vi "SPARK Set Sensor Position.vi"(7 "Sensor (Primary Encoder)":enum16{"Primary Encoder", "Alt/Ext Encoder"}(ring), 8 "error in":errorcluster, 10 "Position":dbl, 11 "MotorControlDeviceRef":T1={"DeviceStatus"={"status"=FALSE, "code"=0, "source"=""}, "Type"=enum."PWM", "PWM"={"PWM Channel"=enum."Invalid", "DeadBand"={"Name"="", "maxPositivePwm"=0, "minPositivePwm"=0, "centerPwm"=0, "maxNegativePwm"=0, "minNegativePwm"=0, "angularRange"=0}}, "CAN"={"Device Number"=0, "SetOutput VI Ref"=variant(refnum<vi> refnum), "GetOutput VI Ref"=variant(refnum<vi> refnum), "Enable VI Ref"=variant(refnum<vi> refnum), "Disable VI Ref"=variant(refnum<vi> refnum), "Data"=variant}, "Invert"=FALSE, "DIO PWM"={"PWM \"Enable\" Channel"=enum."Invalid", "DIOChannel"=enum."Invalid", "PWM Rate"=0.0}}) -> (0 "error out":errorcluster, 3 "MotorControlDeviceRef":T1={"DeviceStatus"={"status"=FALSE, "code"=0, "source"=""}, "Type"=enum."PWM", "PWM"={"PWM Channel"=enum."Invalid", "DeadBand"={"Name"="", "maxPositivePwm"=0, "minPositivePwm"=0, "centerPwm"=0, "maxNegativePwm"=0, "minNegativePwm"=0, "angularRange"=0}}, "CAN"={"Device Number"=0, "SetOutput VI Ref"=variant(refnum<vi> refnum), "GetOutput VI Ref"=variant(refnum<vi> refnum), "Enable VI Ref"=variant(refnum<vi> refnum), "Disable VI Ref"=variant(refnum<vi> refnum), "Data"=variant}, "Invert"=FALSE, "DIO PWM"={"PWM \"Enable\" Channel"=enum."Invalid", "DIOChannel"=enum."Invalid", "PWM Rate"=0.0}})   [LabVIEW 2023]
doc: "Set the position of a sensor. By default the units are 'rotations' and can be changed by a scale factor setting the sensor's position conversion factor."
uses:
  <vilib>/Rock Robotics/WPI/MotorControl/WPI_MotorControlDeviceRef.ctl
  <vilib>/Rock Robotics/WPI/MotorControl/WPI_MotorControlType.ctl
  <vilib>/Rock Robotics/SystemInterfaces/DIO/FPGA_DIOPWMChannel.ctl
  <vilib>/Rock Robotics/WPI/PWM/WPI_PWMDeadband.ctl
  <vilib>/Rock Robotics/SystemInterfaces/DIO/FPGA_DIOChannel.ctl
  Typedef/Spark MAX Variant Data.ctl
  Typedef/SPARK Model.ctl
  Typedef/Spark MAX Parameter Type.ctl
  Typedef/SPARK CAN Arb ID.ctl
  729eceb4-cec2-4d85-8519-0202a9176e1c.vi
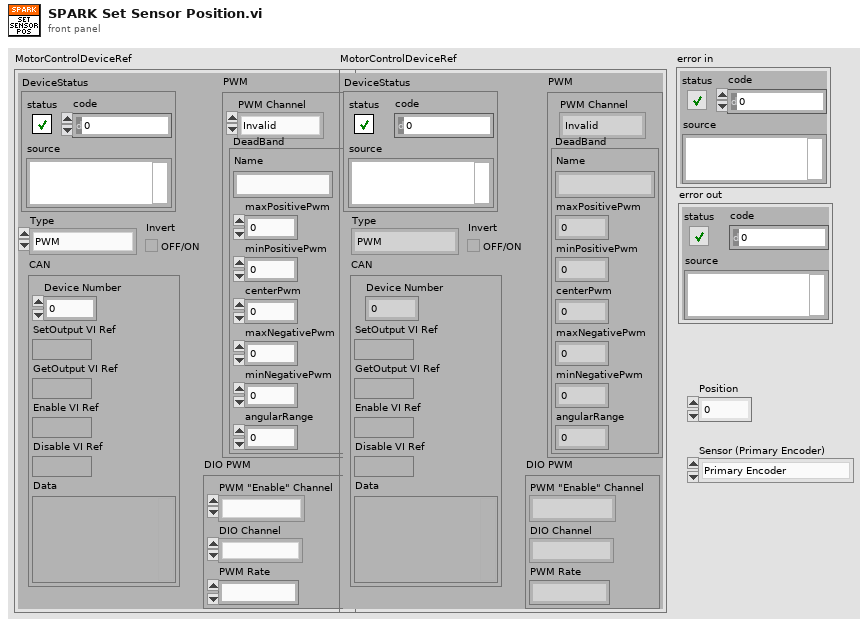
[diagram p1: front panel]
types:
  T1 = typedef "WPI_MotorControlDeviceRef.ctl" = cluster{"DeviceStatus":errorcluster, "Type":T2, "PWM":cluster{"PWM Channel":T3, "DeadBand":T4}, "CAN":cluster{"Device Number":u8, "SetOutput VI Ref":variant, "GetOutput VI Ref":variant, "Enable VI Ref":variant, "Disable VI Ref":variant, "Data":variant}, "Invert":bool, "DIO PWM":cluster{"PWM \"Enable\" Channel":T3, "DIOChannel":T5, "PWM Rate":dbl}}
  T2 = typedef "WPI_MotorControlType.ctl" = enum16{"PWM", "CAN", "DIO PWM"}
  T3 = typedef "FPGA_DIOPWMChannel.ctl" = enum8{"PWM 0", "PWM 1", "PWM 2", "PWM 3", "PWM 4", "PWM 5", "PWM 6", "PWM 7", "PWM 8", "PWM 9", "PWM MXP 0", "PWM MXP 1", "PWM MXP 2", "PWM MXP 3", "PWM MXP 4", "PWM MXP 5", "PWM MXP 6", "PWM MXP 7", "PWM MXP 8", "PWM MXP 9", "Invalid"}
  T4 = typedef "WPI_PWMDeadband.ctl" = cluster{"Name":string, "maxPositivePwm":i32, "minPositivePwm":i32, "centerPwm":i32, "maxNegativePwm":i32, "minNegativePwm":i32, "angularRange":u16}
  T5 = typedef "FPGA_DIOChannel.ctl" = enum8{"DIO 0", "DIO 1", "DIO 2", "DIO 3", "DIO 4", "DIO 5", "DIO 6", "DIO 7", "DIO 8", "DIO 9", "DIO MXP 0", "DIO MXP 1", "DIO MXP 2", "DIO MXP 3", "DIO MXP 4", "DIO MXP 5", "DIO MXP 6", "DIO MXP 7", "DIO MXP 8", "DIO MXP 9", "DIO MXP 10", "DIO MXP 11", "DIO MXP 12", "DIO MXP 13", "DIO MXP 14", "DIO MXP 15", "SPI Port CS1", "SPI Port CS2", "SPI Port CS3", "SPI Port MISO", "SPI Port MOSI", "Invalid"}
  T6 = typedef "Spark MAX Parameter Type.ctl" = enum16{"Unused", "Signed Int", "Unsigned Int", "Float", "Bool"}
  T7 = typedef "Spark MAX Variant Data.ctl" = cluster{"Ext ID":u32, "CAN Timeout":u32, "Inverted No WPILib":bool, "Has Configured Limit Sw":bool, "Has Configured Alt Encoder":bool, "SPARK Model":T8, "CAN Max Retries":u32, "CAN Timeout (ms)":u32, "Status 0 Period (ms)":u32, "Status 1 Period (ms)":u32, "Status 2 Period (ms)":u32, "Status 3 Period (ms)":u32, "Status 4 Period (ms)":u32, "Status 5 Period (ms)":u32, "Status 6 Period (ms)":u32, "Status 7 Period (ms)":u32, "Status Frame Timeout (ms)":u32}
  T8 = typedef "SPARK Model.ctl" = enum16{"SPARK MAX", "SPARK Flex", "Unknown"}
  T9 = typedef "SPARK CAN Arb ID.ctl" = u32
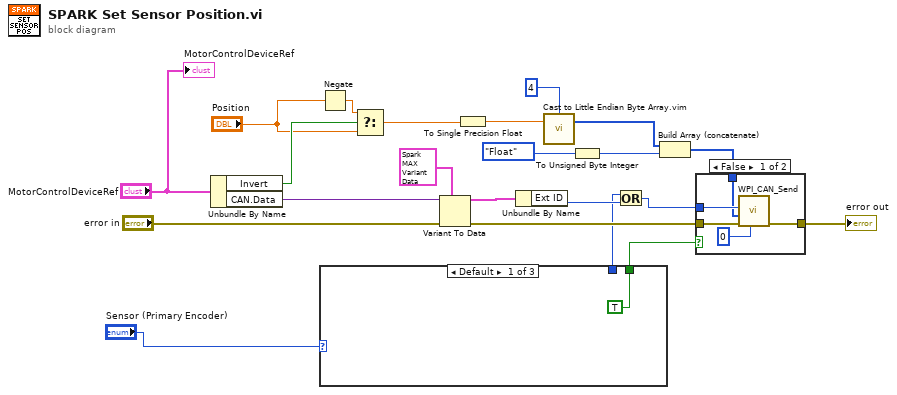
[diagram p0: block diagram]
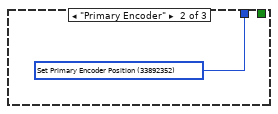
[diagram p3: hidden frame]
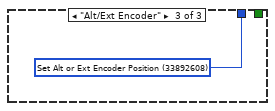
[diagram p4: hidden frame]
diagram:
  n1 = Unbundle By Name("MotorControlDeviceRef") -> ("Invert"=w7:bool, "CAN.Data"=w20:variant)
  n2 = Negate(x="Position") -> (-x=w6:dbl)
  n3 = case shown="Default" "Sensor (Primary Encoder)" {
    tunnel: [_ w24 w25] -> w3
    tunnel: [TRUE _ _] -> w2
    frame Default {
    }
    frame "Primary Encoder" {
      w24 = T9 33892352 items=["Broadcast Disable"=0, "Broadcast System Halt"=64, "Broadcast System Reset"=128, "Broadcast Device Assign"=192, "Broadcast Heartbeat"=320, "Broadcast Firmware Version"=512, "Broadcast Enumerate"=576, "Broadcast System Resume"=640, "Velocity Setpoint"=33882112, "Duty Cycle Setpoint"=33882240, "Smart Velocity Setpoint"=33882304, "Position Setpoint"=33882368, "Voltage Setpoint"=33882432, "Current Setpoint"=33882496, "Smart Motion Setpoint"=33882560, "MAXMotion Position Setpoint"=33882624, "MAXMotion Velocity Setpoint"=33882688, "Periodic Status 0"=33929216, "Periodic Status 1"=33929280, "Periodic Status 2"=33929344, "Periodic Status 3"=33929408, "Periodic Status 4"=33929472, "Periodic Status 5"=33929536, "Periodic Status 6"=33929600, "Periodic Status 7"=33929664, "Set Statuses Enabled"=33883136, "Set Statuses Enabled Response"=33883200, "DRV Status"=33888896, "Clear Faults"=33889152, "Parameter Write"=33896448, "Parameter Write Response"=33896512, "Parameter Double Read Start (RTR)"=33897472, "Persist Parameters"=33947584, "Persist Parameters Response"=33883392, "Reset Parameters"=33883456, "Reset Parameters Response"=33883520, "Set Follower Mode"=33889472, "Nack"=33890304, "Ack"=33890368, "Broadcast (not a command)"=33891328, "Heartbeat"=33891456, "Sync"=33891520, "IDQuery"=33891584, "IDAssign"=33891648, "Get Motor Interface (RTR)"=33894720, "Get Firmware Version (RTR)"=33891840, "REV Enumerate"=33891904, "Legacy/USB Heartbeat"=33891968, "roboRIO Lock"=33892032, "SWDL Data"=33892096, "SWDL Checksum"=33892160, "SWDL Retransmit"=33892224, "Set Primary Encoder Position"=33892352, "Set I Accum"=33892480, "Set Alt or Ext Encoder Position"=33892608, "Non-roboRIO Broadcast (not a command)"=33893376, "non-RIO Lock"=33893440, "Start Follower Mode"=33913856, "Start Follower Mode Response"=33913920, "Stop Follower Mode"=33913984, "Stop Follower Mode Response"=33914048, "non-RIO Heartbeat"=33893504] ("SPARK Arb ID")
    }
    frame "Alt/Ext Encoder" {
      w25 = T9 33892608 items=["Broadcast Disable"=0, "Broadcast System Halt"=64, "Broadcast System Reset"=128, "Broadcast Device Assign"=192, "Broadcast Heartbeat"=320, "Broadcast Firmware Version"=512, "Broadcast Enumerate"=576, "Broadcast System Resume"=640, "Velocity Setpoint"=33882112, "Duty Cycle Setpoint"=33882240, "Smart Velocity Setpoint"=33882304, "Position Setpoint"=33882368, "Voltage Setpoint"=33882432, "Current Setpoint"=33882496, "Smart Motion Setpoint"=33882560, "MAXMotion Position Setpoint"=33882624, "MAXMotion Velocity Setpoint"=33882688, "Periodic Status 0"=33929216, "Periodic Status 1"=33929280, "Periodic Status 2"=33929344, "Periodic Status 3"=33929408, "Periodic Status 4"=33929472, "Periodic Status 5"=33929536, "Periodic Status 6"=33929600, "Periodic Status 7"=33929664, "Set Statuses Enabled"=33883136, "Set Statuses Enabled Response"=33883200, "DRV Status"=33888896, "Clear Faults"=33889152, "Parameter Write"=33896448, "Parameter Write Response"=33896512, "Parameter Double Read Start (RTR)"=33897472, "Persist Parameters"=33947584, "Persist Parameters Response"=33883392, "Reset Parameters"=33883456, "Reset Parameters Response"=33883520, "Set Follower Mode"=33889472, "Nack"=33890304, "Ack"=33890368, "Broadcast (not a command)"=33891328, "Heartbeat"=33891456, "Sync"=33891520, "IDQuery"=33891584, "IDAssign"=33891648, "Get Motor Interface (RTR)"=33894720, "Get Firmware Version (RTR)"=33891840, "REV Enumerate"=33891904, "Legacy/USB Heartbeat"=33891968, "roboRIO Lock"=33892032, "SWDL Data"=33892096, "SWDL Checksum"=33892160, "SWDL Retransmit"=33892224, "Set Primary Encoder Position"=33892352, "Set I Accum"=33892480, "Set Alt or Ext Encoder Position"=33892608, "Non-roboRIO Broadcast (not a command)"=33893376, "non-RIO Lock"=33893440, "Start Follower Mode"=33913856, "Start Follower Mode Response"=33913920, "Stop Follower Mode"=33913984, "Stop Follower Mode Response"=33914048, "non-RIO Heartbeat"=33893504] ("SPARK Arb ID")
    }
  }
  n4 = Select(t=w6, s=w7, f="Position") -> (s? t:f=w4:dbl)
  n5 = Variant To Data(error in="error in", type=T7 {"Ext ID"=0, "CAN Timeout"=0, "Inverted No WPILib"=FALSE, "Has Configured Limit Sw"=FALSE, "Has Configured Alt Encoder"=FALSE, "SPARK Model"=enum."Unknown", "CAN Max Retries"=5, "CAN Timeout (ms)"=20, "Status 0 Period (ms)"=10, "Status 1 Period (ms)"=250, "Status 2 Period (ms)"=20, "Status 3 Period (ms)"=20, "Status 4 Period (ms)"=20, "Status 5 Period (ms)"=20, "Status 6 Period (ms)"=20, "Status 7 Period (ms)"=20, "Status Frame Timeout (ms)"=500}, Variant=w20) -> (data=w18:T7, error out=w16:errorcluster)
  n6 = To Single Precision Float(number=w4) -> (single precision float=w8:sgl)
  n7 = Unbundle By Name(w18) -> ("Ext ID"=w14:u32)
  n8 = call "Cast to Little Endian Byte Array.vim"("value"=w8, "bytes"=4) -> ("output array"=w12:u8[])  [unwired: 1 in]
  n9 = To Unsigned Byte Integer(number=Spark_MAX_Parameter_Type."Float" ("Parameter Type")) -> (unsigned 8bit integer=w9:u8)
  n10 = Or(x=w3, y=w14) -> (x .or. y?=w13:T9)
  n11 = Build Array (concatenate)(w12, w9) -> (w11:u8[])
  n12 = case shown="False" w2 {
    tunnel: w16 -> [w30 w31]
    tunnel: [w29 w31] -> w15
    tunnel: w13 -> [w27 _]
    tunnel: w11 -> [w26 _]
    frame False {
      n13 = call <vilib>:"WPI_CAN_Send.vi"("Period (ms)"=0, "error in (no error)"=w30, "Data"=w26, "Message ID"=w27) -> ("error out"=w29:errorcluster)  [unwired: 7 in]
    }
    frame True {
    }
  }
  "error out" <- w15
  "MotorControlDeviceRef" <- "MotorControlDeviceRef"
